vi "Get Property.vi"(10 "Ctl Ref":refnum<vi>, 11 "UIP In":refnum<class "TemplateUIP.lvclass">) -> (0 "Error Out":errorcluster, 3 "UIP Out":refnum<class "TemplateUIP.lvclass">)   [LabVIEW 2020, in "UIM.lvlib" / "TemplateUIP.lvclass"]
doc: "Modify this method to implement functionality for extracting the property from VI Server Control to be stored inside UIP."
uses:
  TemplateUIP.lvclass
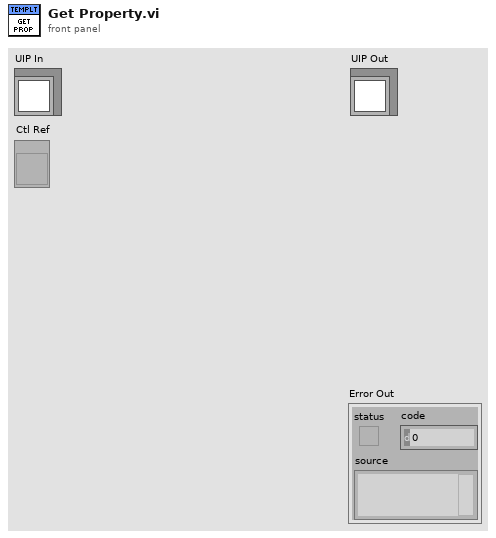
[diagram p1: front panel]
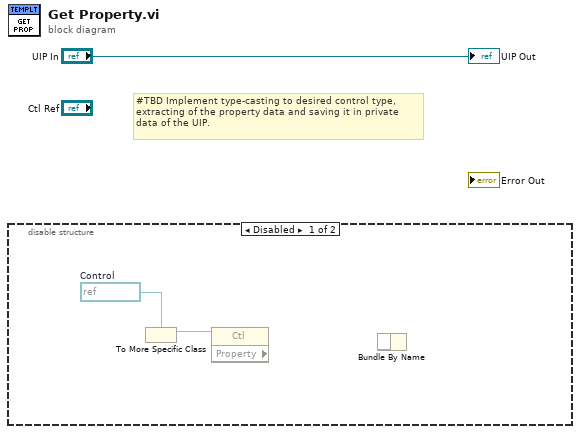
[diagram p0: block diagram]
diagram:
  # "#TBD Implement type-casting to desired control type,\nextracting of the property data and saving it in private \ndata of the UIP."
  n1 = disable-structure shown="Disabled" {
    frame Disabled {
      w3 = refnum<vi> refnum  # Control
      n2 = To More Specific Class(target class=w3) -> (specific class reference=w2:refnum<vi>)  [unwired: 2 in, 1 out]
      n3 = property class="Ctl" props=[](reference=w2) -> ()  [unwired: 1 in, 3 out]
      n4 = Bundle By Name "Bundle By Name"() -> ()  [unwired: 2 in, 1 out]
    }
    frame Enabled {
    }
  }
  "UIP Out" <- "UIP In"
